vi "Configure Scanning.vi"(6 "Channel 2 Readings (1)":i32=1, 7 "External Scan List ((@1:10))":string="(@1:10)", 8 "error in (no error)":errorcluster, 9 "Channel 1 Readings (1)":i32=1, 10 "Enable Scanning (0: None)":i32(ring) items=["None", "Internal", "External"], 11 "VISA resource name":refnum<visa-resource-name>) -> (0 "error out":errorcluster, 3 "VISA resource name out":refnum<visa-resource-name>)   [LabVIEW 2021, in "Keithley 2182.lvlib"]
doc: "Configures internal and extern scanning settings.\n\nThe Model 2182 can step or scan its two input channels or be used with external scanner cards\ninstalled in switching mainframes such as Models 707, 7001, and 7002"
uses:
  <instrlib>/Keithley 2182/Keithley 2182.lvlib
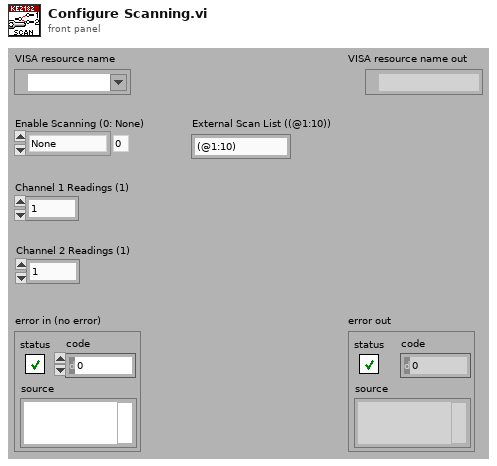
[diagram p1: front panel]
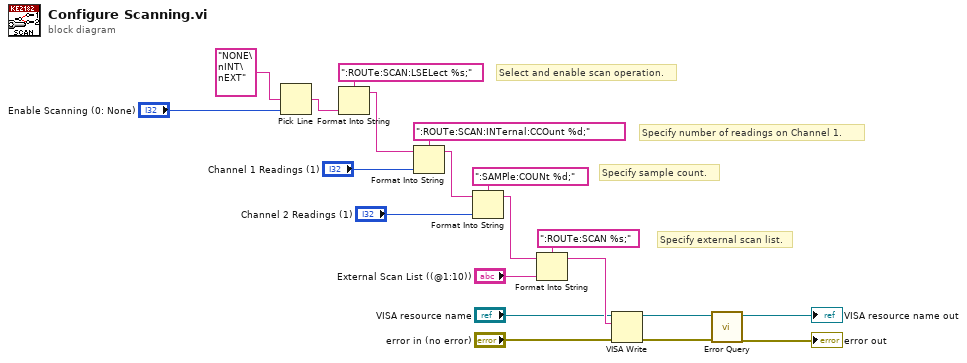
[diagram p0: block diagram]
diagram:
  # "Specify external scan list."
  # "Specify number of readings on Channel 1."
  # "Select and enable scan operation."
  # "Specify sample count."
  n1 = Pick Line(multi-line string="NONE\nINT\nEXT", line index="Enable Scanning (0: None)") -> (output string=w7:string)  [unwired: 1 in]
  n2 = Format Into String(format string=":ROUTe:SCAN:LSELect %s;", w7) -> (resulting string=w19:string)  [unwired: 2 in, 1 out]
  n3 = Format Into String(format string=":ROUTe:SCAN:INTernal:CCOunt %d;", initial string=w19, "Channel 1 Readings (1)") -> (resulting string=w3:string)  [unwired: 1 in, 1 out]
  n4 = Format Into String(format string=":SAMPle:COUNt %d;", initial string=w3, "Channel 2 Readings (1)") -> (resulting string=w2:string)  [unwired: 1 in, 1 out]
  n5 = Format Into String(format string=":ROUTe:SCAN %s;", initial string=w2, "External Scan List ((@1:10))") -> (resulting string=w14:string)  [unwired: 1 in, 1 out]
  n6 = VISA Write(VISA resource name="VISA resource name", write buffer=w14, error in (no error)="error in (no error)") -> (VISA resource name out=w11:refnum<visa-resource-name>, error out=w10:errorcluster)  [unwired: 1 out]
  n7 = call <instrlib>:"Error Query.vi"("error in (no error)"=w10, "VISA resource name"=w11) -> ("error out"=→"error out":errorcluster, "VISA resource name out"=→"VISA resource name out":refnum<visa-resource-name>)  [unwired: 6 in, 2 out]
